vi "GetButtonNumber.vi"(8 "Error In":errorcluster, 11 "BTN Ref In":refnum<vi>) -> (0 "Error Out":errorcluster, 3 "BTN Nr Out":string)   [LabVIEW 2011]
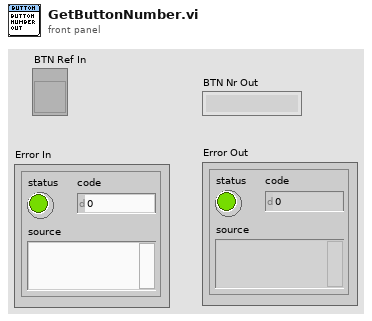
[diagram p1: front panel]
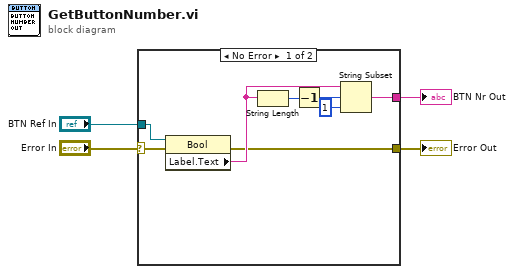
[diagram p0: block diagram]
diagram:
  n1 = case shown="No Error" "Error In" {
    selector: "Error In" -> [w5 w13]
    tunnel: [w12 _] -> w4
    tunnel: "BTN Ref In" -> [w7 _]
    tunnel: [w6 w13] -> w2
    frame No Error {
      n2 = property class="Bool"(reference=w7, error in=w5) -> (error out=w6:errorcluster, "Label.Text"=w9:string)  [unwired: 1 out]
      n3 = String Length(string=w9) -> (length=w10:i32)
      n4 = Decrement(x=w10) -> (x-1=w11:i32)
      n5 = String Subset(string=w9, offset (0)=w11, length (rest)=1 ("length (rest)")) -> (substring=w12:string)
    }
    frame Error {
    }
  }
  "BTN Nr Out" <- w4
  "Error Out" <- w2
